vi "Init RS232.vi"(11 "Error IN":errorcluster) -> (4 "FPGA Main Reference Out":refnum<k20>, 15 "error out":errorcluster)   [LabVIEW 2011]
uses:
  <vilib>/rvi/interface/nirviOpenFPGA/nirviOpenFPGA.xnode
  <vilib>/rvi/interface/nirviMethod/nirviMethod.xnode
  FPGA Source/FPGA Main.vi
  FPGA Bitfiles/JAGM_FPGATarget_FPGAMain_3783B04E.lvbitx
  <vilib>/FPGAPlugInAG/sbRIO-9606/niLvFpga_Open_sbRIO-9606.vi
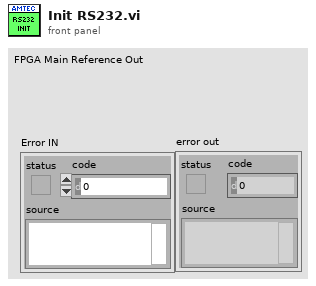
[diagram p1: front panel]
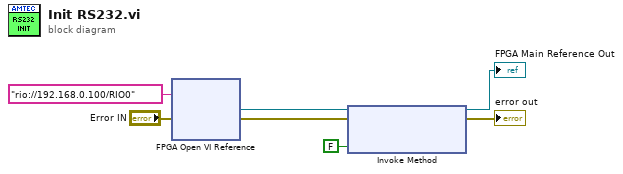
[diagram p0: block diagram]
diagram:
  n1 = xnode "FPGA Open VI Reference"("error in"="Error IN", "resource name"=tag "rio://192.168.0.100/RIO0") -> ("FPGA VI Reference Out"=w3:refnum<k20>, "error out"=w4:errorcluster)
  n2 = xnode "Invoke Method"("FPGA VI Reference In"=w3, "error in"=w4, "Wait Until Done (F)"=FALSE) -> ("FPGA VI Reference Out"=→"FPGA Main Reference Out":refnum<k20>, "error out"=→"error out":errorcluster)
